vi "waitTrigger.vi"(8 "error in (no error)":errorcluster, 9 "timeout (ms) default: 10s":i32, 10 "IRQ":i32, 11 "Refnum in":refnum<k20>) -> (0 "error out":errorcluster, 1 "Boolean":bool, 2 "Timed Out":bool, 3 "Refnum out":refnum<k20>)   [LabVIEW 2014]
uses:
  <vilib>/Utility/error.llb/Error Cluster From Error Code.vi
  <vilib>/RVI Host/nirviSupport.llb/nirviErrorClusterFromErrorCode.vi
  <vilib>/rvi/errors/niLvFpgaAdjustHostInterfaceError.vi
  <vilib>/rvi/interface/nirviMethod/nirviMethod.xnode
  FPGA Bitfiles/W7XBolo2017_FPGATarget_fmain2014_9xlV3GyHFfo.lvbitx
  f_main_2014.vi
  <vilib>/rvi/interface/nirviMethod/StockFPGA_InlinedMethodWaitForSingleIRQ.vi
  <vilib>/FPGAPlugInAG/PCI-7813R/niLvFpga_WaitOnIrq_PCI-7813R.vi
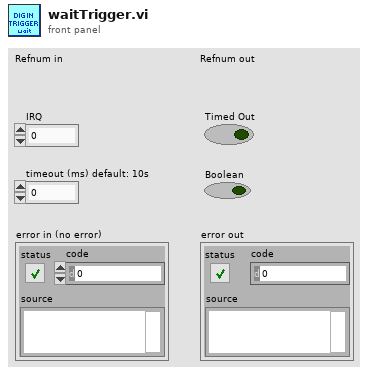
[diagram p1: front panel]
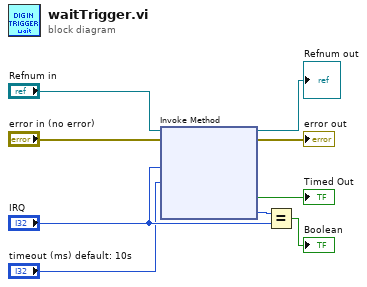
[diagram p0: block diagram]
diagram:
  n1 = xnode "Invoke Method"("FPGA VI Reference In"="Refnum in", "error in"="error in (no error)", "IRQ Number(s)"="IRQ", "Timeout (ms)"="timeout (ms) default: 10s") -> ("FPGA VI Reference Out"=→"Refnum out":refnum<k20>, "error out"=→"error out":errorcluster, "Timed Out"=→"Timed Out":bool, "IRQ(s) Asserted"=w6:i32)
  n2 = Equal?(x=w6, y="IRQ") -> (x = y?=→"Boolean":bool)
